vi "多参数数据插入.vi"(8 "error in (no error)":errorcluster caption="错误输入（无错误）", 9 "编号":string, 10 "columns enable":T1, 11 "data in":T2) -> (0 "error out":errorcluster)   [LabVIEW 2016, in "斯坦道原位多参数.lvlib"]
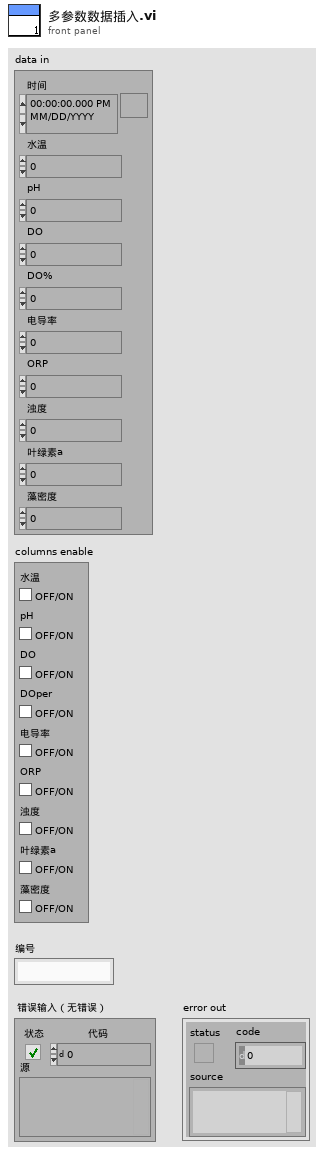
[diagram p1: front panel]
types:
  T1 = cluster{"水温":bool, "pH":bool, "DO":bool, "DOper":bool, "电导率":bool, "ORP":bool, "浊度":bool, "叶绿素a":bool, "藻密度":bool}
  T2 = typedef "原位多参数全参数字段定义.ctl" = cluster{"时间":timestamp, "水温":dbl, "pH":dbl, "DO":dbl, "DO%":dbl, "电导率":dbl, "ORP":dbl, "浊度":dbl, "叶绿素a":dbl, "藻密度":dbl}
  T3 = cluster{"columns外部输入":bool, "columns input":string[]}
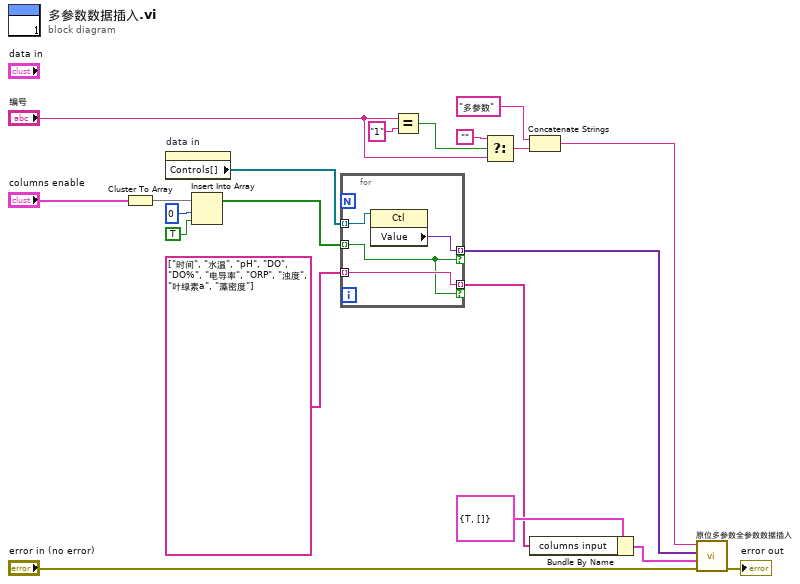
[diagram p0: block diagram]
diagram:
  n1 = Cluster To Array(cluster="columns enable") -> (array=w13:bool[])
  n2 = property on="data in" class="Clust (严格)"() -> ("Controls[]"=w15:refnum<vi>[])  [unwired: 2 in, 2 out]
  n3 = Insert Into Array(array=w13, index=0 ("索引"), new element=TRUE ("新元素/子数组")) -> (w14:bool[])
  n4 = for {
    tunnel: w15 -> [w24] mode=indexing
    tunnel: [w23] -> w5 mode=indexing if=w21
    tunnel: string[] ["时间", "水温", "pH", "DO", "DO%", "电导率", "ORP", "浊度", "叶绿素a", "藻密度"] -> [w22] mode=indexing
    tunnel: [w22] -> w8 mode=indexing if=w21
    tunnel: w14 -> [w21] mode=indexing
    n5 = property class="Ctl"(reference=w24) -> ("Value"=w23:variant)  [unwired: 1 in, 2 out]
  }
  n6 = Equal?(x="编号", y="1") -> (x = y?=w18:bool)
  n7 = Select(t="", s=w18, f="编号") -> (s? t:f=w16:string)
  n8 = Concatenate Strings("多参数" ("字符串"), w16) -> (w6:string)
  n9 = Bundle By Name(cluster=T3 {"columns外部输入"=TRUE, "columns input"=[]} ("columns外部输入"), "columns input"=w8) -> (w4:T3)
  n10 = call "原位多参数全参数数据插入.vi"("Tabe Name"=w6, "data"=w5, "columns外部输入"=w4, "错误输入（无错误）"="error in (no error)") -> ("错误输出"=→"error out":errorcluster)  [unwired: 6 in]
